vi "Read Stderr.vi"(8 "Error In":errorcluster, 10 "Max Data Length":i32=1024 min=0 max=30000, 11 "Channel In":refnum<class "Channel.lvclass">) -> (0 "Error Out":errorcluster, 2 "Data":u8[](array[numeric]), 3 "Channel Out":refnum<class "Channel.lvclass">)   [LabVIEW 2021, in "Field_RnD_Services_LIBSSH2_Toolkit.lvlib" / "Channel.lvclass"]
doc: "Reads binary data from the remote SSH server's STDERR stream through the SSH channel represented by this Channel object. The <B>Max Data Length</B> must be greater than or equal to the expected data that is returned from the remote SSH server to avoid an error. Note, there is a hard-coded maximum of 30KB in the libssh2 shared library. If the expected data is greater than 30KB, then this VI should be executed in a loop that accummlates the <B>Data</B> array size for each execution and stops when the total binary data size has been reached."
uses:
  Channel.lvclass
  Session/Session.lvclass
  Field_RnD_Services_LIBSSH2_Toolkit.lvlib
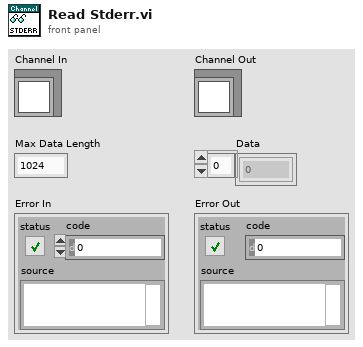
[diagram p1: front panel]
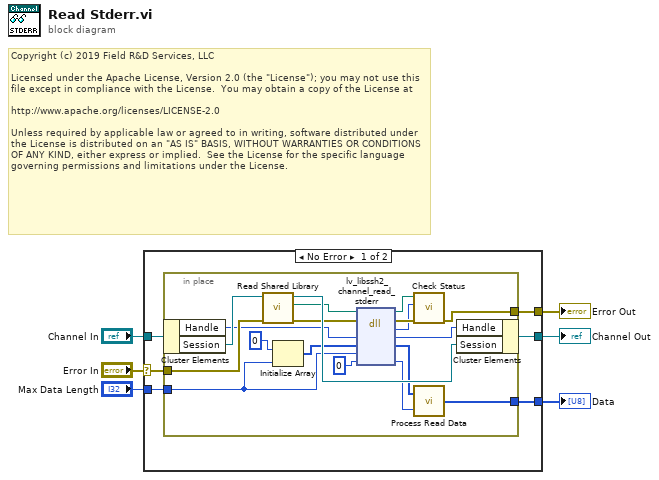
[diagram p0: block diagram]
diagram:
  # "Copyright (c) 2019 Field R&D Services, LLC\n\nLicensed under the Apache License, Version 2.0 (the \"License\"); you may not use this file except in compliance with the License.  You may obtain a copy of the License at\n\nhttp://www.apache.org/licenses/LICENSE-2.0\n\nUnless required by applicable law or agreed to in writing, software distributed under the License is distributed on an \"AS IS\" BASIS, WITHOUT WARRANTIES OR CONDITIONS OF ANY KIND, either express or implied.  See the License for the specific language governing permissions and limitations under the License."
  n1 = case shown="No Error" "Error In" {
    selector: "Error In" -> [w10 w32]
    tunnel: [w9 w32] -> w5
    tunnel: "Channel In" -> [w12 w31]
    tunnel: [w11 w31] -> w3
    tunnel: "Max Data Length" -> [w8 _]
    tunnel: [w7 _] -> w1
    frame No Error {
      n2 = in-place {
        in-place-border: w10 -> [w26]
        in-place-border: [w22] -> w9
        in-place-border: w8 -> [w16]
        in-place-border: [w14] -> w7
        n3 = in-place-cluster #1(w12) -> ("Handle"=w21:u64, "Session"=w30:refnum<class "Session.lvclass">)
        n4 = call "Read Shared Library.vi"("Error In"=w26, "Session In"=w30) -> ("Erorr Out"=w27:errorcluster, "libssh2lv Shared Library"=w28:path, "Session Out"=w29:refnum<class "Session.lvclass">)  [unwired: 7 in]
        n5 = Initialize Array(u8 0, w16) -> (w19:u8[])
        n6 = dll-call lib="libssh2lv.*" fn="lv_libssh2_channel_read_stderr"(path in=w28, error in=w27, "handle"=w21, "buffer"=w19, "buffer_len"=w16, "byte_count"=u64 0) -> (path out=w24:path, error out=w25:errorcluster, "status"=w23:i32, "handle"=w20:u64, "buffer"=w15:u8[], "byte_count"=w13:u64)  [unwired: 2 in]
        n7 = call "Check Status.vi"("Error In"=w25, "Status"=w23, "libssh2lv Shared Library In"=w24) -> ("Error Out"=w22:errorcluster)  [unwired: 7 in, 1 out]
        n8 = call "Process Read Data.vi"("Bytes Read Count"=w13, "Data In"=w15) -> ("Data Out"=w14:u8[])
        n9 = in-place-cluster #1("Handle"=w20, "Session"=w29) -> (w11:refnum<class "Channel.lvclass">)
      }
    }
    frame Error {
    }
  }
  "Error Out" <- w5
  "Channel Out" <- w3
  "Data" <- w1
